vi "Configure Scheduled Tx Channel.vi"(8 "error in":errorcluster, 9 "labels settings for RT":T1[](array[typedef]) {"Label Timestamp Channel Data Reference" format="%.0x"; "Word Initial Raw Value" format="%032.0f"; "Label Disable/Trigger Channel Reference" format="%.0x"; "parameter driver data"."Tx parameter refs" format="%.0x"; "SDI" format="%02b"; "label" format="%.0o"}, 10 "channel number in":u8, 11 "board handle in":u8) -> (0 "error out":errorcluster, 2 "channel number out":u8, 3 "board handle out":u8)   [LabVIEW 2020, in "AIM ARINC 429 Hardware API.lvlib"]
doc: "Configures all of the labels for a specified channel to be received."
uses:
  AIM ARINC 429 Hardware API.lvlib
  <instrlib>/AIM GmbH/_ARINC-429/AIM429LV.lvlib
  Shared/Label.ctl
  <vilib>/NI/NI VeriStand Encoding and Decoding/Encoding.ctl
  <vilib>/NI/NI VeriStand Encoding and Decoding/Encoding and Decoding.lvlib
  Shared/Parameter Definition.ctl
  <vilib>/NI VeriStand/Custom Device API/Custom Device Item Ref.ctl
  <vilib>/NI VeriStand/Custom Device API/Custom Device API.lvlib
  Shared/RT Parameters.ctl
  Shared/Transfer Type.ctl
  <vilib>/NI VeriStand/Custom Device API/Data Reference.ctl
  Shared/RT Label Settings.ctl
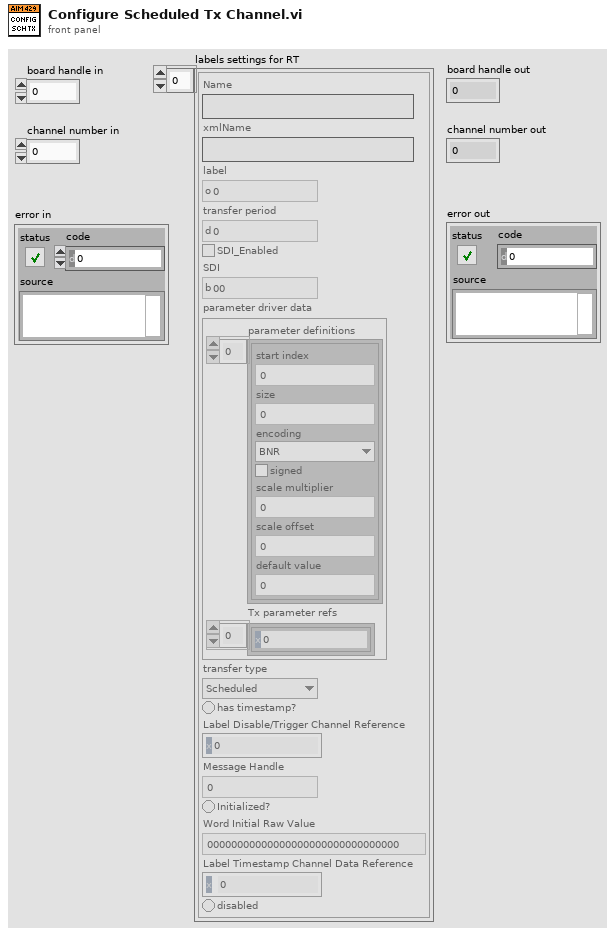
[diagram p1: front panel]
types:
  T1 = typedef "RT Label Settings.ctl" = cluster{"Name":string, "xmlName":string, "label":T2, "transfer period":u32, "SDI_Enabled":bool, "SDI":u8, "parameter driver data":T3, "transfer type":T7, "has timestamp?":bool, "Label Disable/Trigger Channel Reference":T6, "Message Handle":u64, "Initialized?":bool, "Word Initial Raw Value":u32, "Label Timestamp Channel Data Reference":T8, "disabled":bool}
  T2 = typedef "Label.ctl" = u8
  T3 = typedef "RT Parameters.ctl" = cluster{"parameter definitions":T4[], "Tx parameter refs":T6[]}
  T4 = typedef "Parameter Definition.ctl" = cluster{"start index":i32, "size":i32, "encoding":T5, "signed":bool, "scale multiplier":dbl, "scale offset":dbl, "default value":dbl}
  T5 = typedef "Encoding and Decoding.lvlib/Encoding.ctl" = enum16{"BNR", "BCD", "Discrete"}
  T6 = typedef "Custom Device API.lvlib/Custom Device Item Ref.ctl" = u64
  T7 = typedef "Transfer Type.ctl" = enum16{"Scheduled", "Acyclic", "Block", "Strobe"}
  T8 = typedef "Custom Device API.lvlib/Data Reference.ctl" = i32
  T9 = cluster{"xfer_id":u32, "xfer_type":u32, "err_type":u32, "xfer_gap":u16, "ir_index":u16, "buf_size":u16, "xfer_ir":u8}
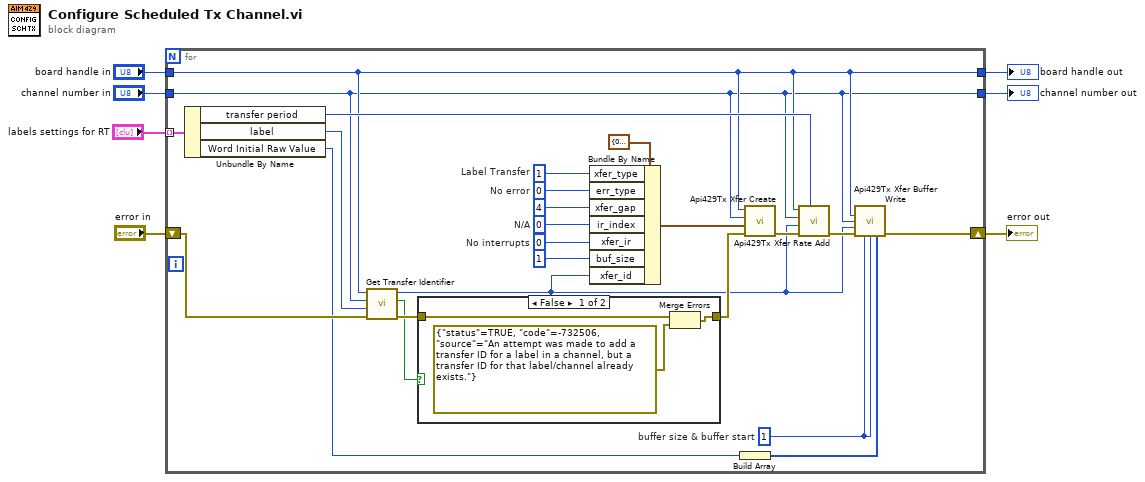
[diagram p0: block diagram]
diagram:
  n1 = for {
    tunnel: "channel number in" -> [w20]
    shift-right: [w13] -> w5
    shift-left: "error in" -> [w31]
    tunnel: "labels settings for RT" -> [w24] mode=indexing
    tunnel: [w20] -> w3
    tunnel: "board handle in" -> [w21]
    tunnel: [w21] -> w1
    w10 = u16 1  # buffer size & buffer start
    w25 = u8 0  # No interrupts
    w27 = u16 0  # N/A
    w29 = u32 0  # No error
    w30 = u32 1  # Label Transfer
    n2 = Unbundle By Name(w24) -> ("transfer period"=w23:u32, "label"=w17:T2, "Word Initial Raw Value"=w18:u32)
    n3 = call "Get Transfer Identifier.vi"("error in"=w31, "label number in"=w17, "channel number in"=w20, "board number in"=w21) -> ("error out"=w19:errorcluster, "new entry created"=w11:bool, "Transfer ID out"=w12:u32)  [unwired: 5 in]
    n4 = case shown="False" w11 {
      tunnel: w19 -> [w34 w35]
      tunnel: [w33 w35] -> w16
      frame False {
        n5 = Merge Errors(w34, errorcluster {"status"=TRUE, "code"=-732506, "source"="An attempt was made to add a transfer ID for a label in a channel, but a transfer ID for that label/channel already exists."} ("error constant")) -> (w33:errorcluster)
      }
      frame True {
      }
    }
    n6 = Bundle By Name(cluster=T9 {"xfer_id"=0, "xfer_type"=1, "err_type"=0, "xfer_gap"=0, "ir_index"=0, "buf_size"=0, "xfer_ir"=0} ("px_Xfer"), "xfer_type"=w30, "err_type"=w29, "xfer_gap"=u16 4 ("transfer gap in bits"), "ir_index"=w27, "xfer_ir"=w25, "buf_size"=u16 1 ("buffer size"), "xfer_id"=w12) -> (w9:T9)
    n7 = Build Array(w18) -> (w22:u32[])
    n8 = call <instrlib>:"Api429Tx Xfer Create.vi"("error in (no error)"=w16, "px_Xfer"=w9, "b_Chn"=w20, "board_handle"=w21) -> ("error out"=w15:errorcluster)  [unwired: 6 in, 1 out]
    n9 = call <instrlib>:"Api429Tx Xfer Rate Add.vi"("ulRateInMs"=w23, "error in (no error)"=w15, "ulXferId"=w12, "ucChannel"=w20, "board_handle"=w21) -> ("error out"=w14:errorcluster)  [unwired: 6 in]
    n10 = call <instrlib>:"Api429Tx Xfer Buffer Write.vi"("board_handle"=w21, "b_Chn"=w20, "ul_XferId"=w12, "error in (no error)"=w14, "w_BufStart"=w10, "w_BufSize"=w10, "pl_LData"=w22) -> ("error out"=w13:errorcluster)  [unwired: 8 in]
  }
  "board handle out" <- w1
  "channel number out" <- w3
  "error out" <- w5
